vi "Blobs.vi"(8 "error in (no error)":errorcluster caption="entrée d'erreur (pas d'erreur)", 11 "make_blobs":T2={"n_samples"=[100], "n_features"=2, "centers"=[], "cluster_std"=[1.0], "centermin"=-10.0, "centermax"=10.0, "shuffle"=TRUE, "random_state"=-1, "Returns"="X"} {"random_state" min=-1; "n_features" min=1}) -> (0 "error out":errorcluster, 3 "Data":T1)   [LabVIEW 2020]
doc: "Generate isotropic Gaussian blobs for clustering.\nProvides greater control regarding the centers and standard deviations of each cluster, and is used to demonstrate clustering\n\nParameters :\n\n- n_samples : int or array-like, optional (default=100)\nIf int, it is the total number of points equally divided among clusters. If array-like, each element of the sequence indicates the number of samples per cluster.\n\n- n_features : int, optional (default=2)\nThe number of features for each sample.\n\n- centers : int or array of shape [n_centers, n_features], optional\n(default=None) The number of centers to generate, or the fixed center locations. If n_samples is an int and centers is None, 3 centers are generated. If n_samples is array-like, centers must be either None or an array of length equal to the length of n_samples.\n\n- cluster_std : float or sequence of floats, optional (default=1.0)\nThe standard deviation of the clusters.\n\n-center_box : pair of floats (min, max), optional (default=(-10.0, 10.0))\nThe bounding box for each cluster center when centers are generated at random.\n\n- shuffle : boolean, optional (default=True)\nShuffle the samples.\n\n- random_state : int, RandomState instance, default=None=-1\nDetermines random number generation for dataset creation. Pass an int for reproducible output across multiple function calls. See Glossary.\n\n\nReturns :\n\n- X : array of shape [n_samples, n_features]\nThe generated samples.\n\n- y array of shape [n_samples]\nThe integer labels for cluster membership of each sample.\n\n- centers : array, shape [n_centers, n_features]\nThe centers of each cluster. Only returned if return_centers=True."
uses:
  Blobs.lvclass
panel:
  out "Blobs.lvclass":refnum<class "Blobs.lvclass">
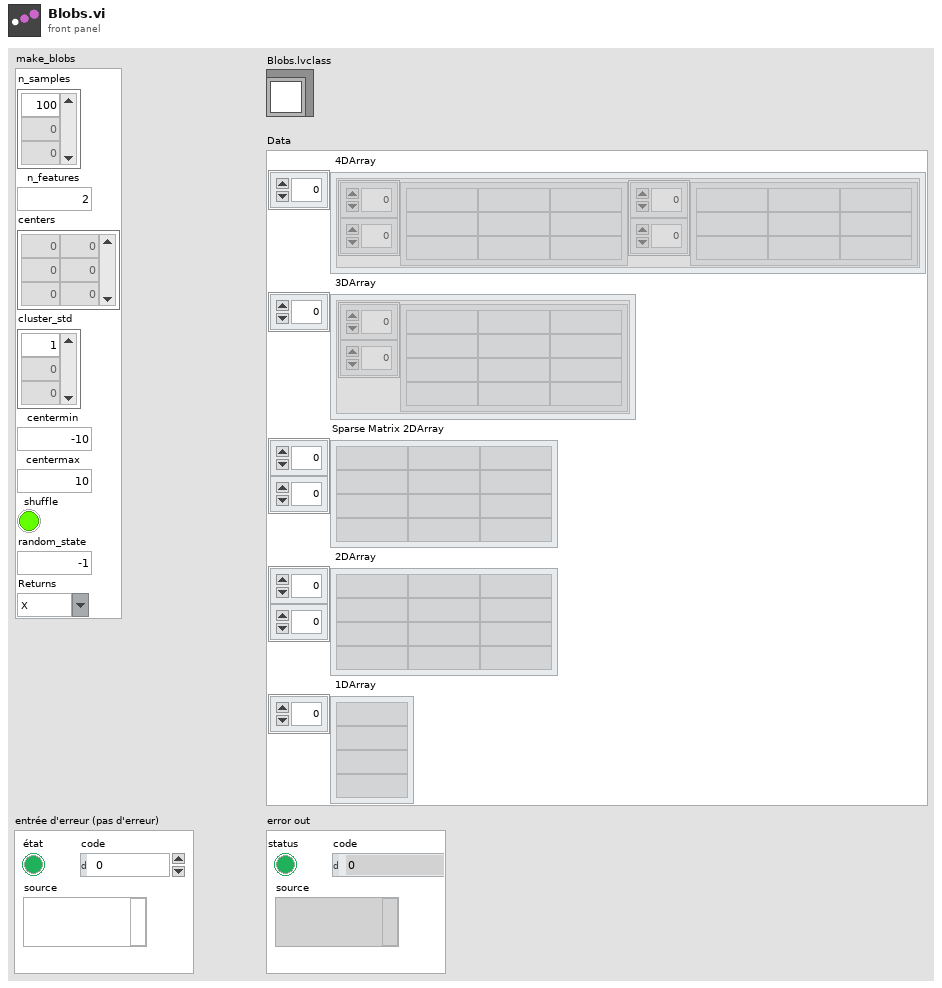
[diagram p1: front panel]
types:
  T1 = cluster{" 4DArray":cluster{"1":string[][], "2":string[][]}[], " 3DArray":cluster{"Tableau":string[][]}[], "Sparse Matrix 2DArray":string[][], " 2DArray":string[][], " 1DArray":string[]}
  T2 = cluster{"n_samples":i32[], "n_features":u32, "centers":i32[][], "cluster_std":dbl[], "centermin":dbl, "centermax":dbl, "shuffle":bool, "random_state":i32, "Returns":string}
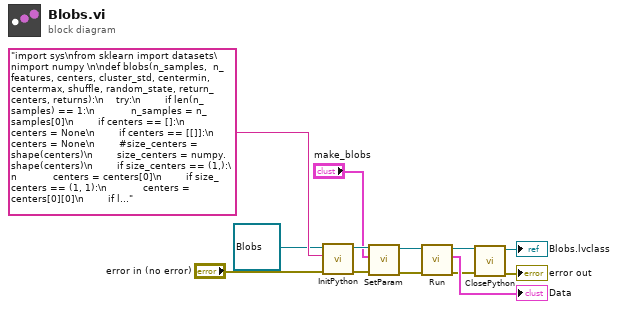
[diagram p0: block diagram]
diagram:
  n1 = call-dynamic "InitPython.vi"("error in (no error)"="error in (no error)", "Python Instruction"="import sys\nfrom sklearn import datasets\nimport numpy \n\ndef blobs(n_samples,  n_features, centers, cluster_std, centermin, centermax, shuffle, random_state, return_centers, returns):\n    try:\n        if len(n_samples) == 1:\n            n_samples = n_samples[0]\n        if centers == []:\n            centers = None\n        if centers == [[]]:\n            centers = None\n        #size_centers = shape(centers)\n        size_centers = numpy.shape(centers)\n        if size_centers == (1,):\n            centers = centers[0]\n        if size_centers == (1, 1):\n            centers = centers[0][0]\n        if len(cluster_std) == 1:\n           cluster_std = cluster_std[0]\n        if random_state == -1:\n            random_state = None\n        X, y, centers = datasets.make_blobs(n_samples,  n_features, centers, cluster_std, (centermin, centermax), shuffle, random_state, return_centers)\n        if returns == 'X':\n            dataX = X.tolist()\n            return str(dataX)\n        elif returns == 'Y' :\n            data_y = y.tolist()\n            return str(data_y)\n        else:\n            data_centers = centers.tolist()\n            return str(data_centers)\n    except:\n        erreur = sys.exc_info()\n        typerr = u\"%s\" % (erreur[0])\n        typerr = typerr[typerr.find(\"'\")+1:typerr.rfind(\"'\")]\n        msgerr = u\"%s\" % (erreur[1])\n        message = str('/!\\\\ {0} : {1}'. format(typerr,msgerr))\n        return message", "Scikit-learn en entrée"=refnum<class "Blobs.lvclass"> refnum ("Blobs.lvclass")) -> ("error out"=w9:errorcluster, "Scikit-learn en sortie"=w10:refnum<class "Blobs.lvclass">)  [unwired: 7 in]
  n2 = call-dynamic "SetParam.vi"("error in (no error)"=w9, "make_blobs"="make_blobs", "Blobs.lvclass"=w10) -> ("error out"=w6:errorcluster, "Blobs.lvclass"=w7:refnum<class "Blobs.lvclass">)  [unwired: 7 in]
  n3 = call-dynamic "Run.vi"("error in (no error)"=w6, "Blobs.lvclass"=w7) -> ("error out"=w3:errorcluster, "Data"=→"Data":T1, "Blobs.lvclass"=w5:refnum<class "Blobs.lvclass">)  [unwired: 7 in]
  n4 = call-dynamic "ClosePython.vi"("error in (no error)"=w3, "Scikit-learn en entrée"=w5) -> ("error out"=→"error out":errorcluster, "Scikit-learn en sortie"=→"Blobs.lvclass":refnum<class "Blobs.lvclass">)  [unwired: 8 in]
